vi "Flush.vi"(8 "error in (no error)":errorcluster, 9 "buffer size":i32=70, 10 "Iterations":i32=2, 11 "VISA resource name":refnum<visa-resource-name>) -> (0 "error out":errorcluster, 3 "VISA resource name out":refnum<visa-resource-name>)   [LabVIEW 2014, in "Hokuyo URG Series.lvlib"]
doc: "This VI does <b>iterations</b> number of VISA reads with each read having a buffer size of <b>buffer size</b>. This is done primarily to flush the buffer."
uses:
  Hokuyo URG Series.lvlib
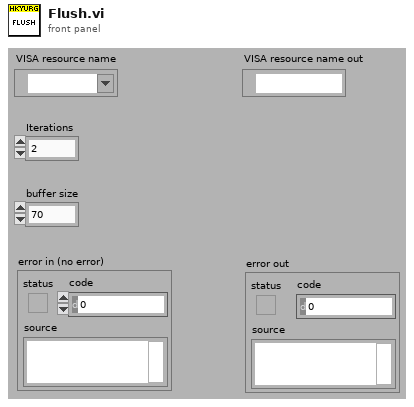
[diagram p1: front panel]
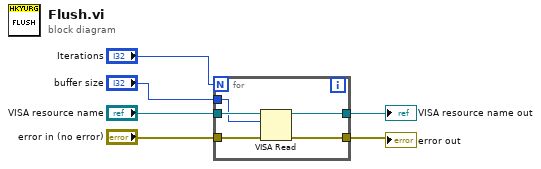
[diagram p0: block diagram]
diagram:
  n1 = for {
    N: "Iterations" -> [_]
    tunnel: [w11] -> w4
    tunnel: [w10] -> w3
    tunnel: "VISA resource name" -> [w9]
    tunnel: "error in (no error)" -> [w8]
    tunnel: "buffer size" -> [w7]
    n2 = VISA Read(VISA resource name=w9, byte count=w7, error in (no error)=w8) -> (VISA resource name out=w11:refnum<visa-resource-name>, error out=w10:errorcluster)  [unwired: 2 out]
  }
  "VISA resource name out" <- w4
  "error out" <- w3
